vi "replace top level section in TOML data.vi"(7 "Section name":string caption="Section name (Section data name if empty)", 8 "error in (no error)":errorcluster, 10 "Section data":variant, 11 "Value in":T1) -> (0 "error out":errorcluster, 3 "Value out":T1)   [LabVIEW 2017, in "TOML.lvlib"]
doc: "Edit a top level element (section) in the TOML data\nMatch the elemnt by \"Section name\""
uses:
  TOML.lvlib
  TOML Value.ctl
  TOML Key-Value Pair.ctl
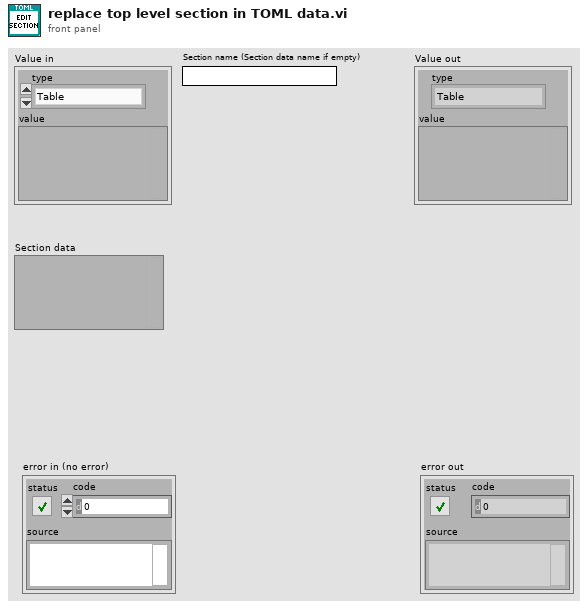
[diagram p1: front panel]
types:
  T1 = typedef "TOML.lvlib/TOML Value.ctl" = cluster{"type":enum16{"Table", "Array", "String", "Integer", "Float", "Boolean", "Offset Date-Time", "Local Date-Time", "Local Date", "Local Time", "Path"}, "value":variant}
  T2 = typedef "TOML.lvlib/TOML Key-Value Pair.ctl" = cluster{"Key":string, "Value":T1}
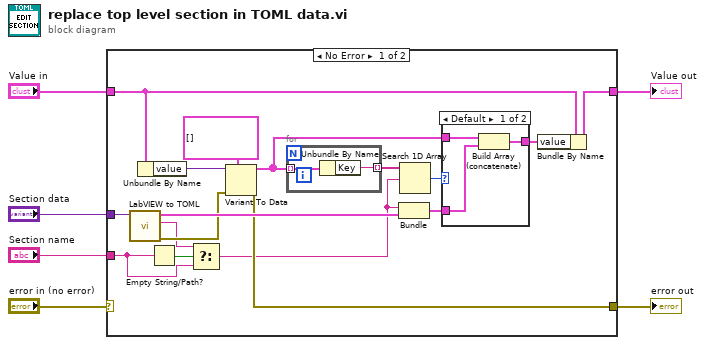
[diagram p0: block diagram]
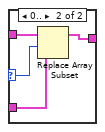
[diagram p2: hidden frame]
diagram:
  n1 = case shown="No Error" "error in (no error)" {
    selector: "error in (no error)" -> [_ w34]
    tunnel: [w22 w33] -> w6
    tunnel: "Value in" -> [w21 w33]
    tunnel: "Section data" -> [w13 _]
    tunnel: "Section name" -> [w8 _]
    tunnel: [w12 w34] -> w1
    frame No Error {
      n2 = call "LabVIEW to TOML.vi"("LV Value"=w13) -> ("error out"=w11:errorcluster, "Name"=w9:string, "TOML Value"=w19:T1)  [unwired: 8 in]
      n3 = Unbundle By Name(w21) -> ("value"=w20:variant)
      n4 = Empty String/Path?(string/path=w8) -> (empty?=w10:bool)
      n5 = Select(t=w9, s=w10, f=w8) -> (s? t:f=w7:string)
      n6 = Variant To Data(error in=w11, type=T2[] [], Variant=w20) -> (data=w16:T2[], error out=w12:errorcluster)
      n7 = for {
        tunnel: w16 -> [w32] mode=indexing
        tunnel: [w31] -> w17 mode=indexing
        n8 = Unbundle By Name(w32) -> ("Key"=w31:string)
      }
      n9 = Bundle("Section name"=w7, "TOML Value"=w19) -> (w15:cluster{"Section name":string, "TOML Value":T1})  [unwired: 1 in]
      n10 = Search 1D Array(1D array=w17, element=w7) -> (index of element=w14:i32)  [unwired: 1 in]
      n11 = case shown="Default" w14 {
        selector: w14 -> [_ w29]
        tunnel: w16 -> [w26 w30]
        tunnel: [w25 w28] -> w23
        tunnel: w15 -> [w24 w27]
        frame Default {
          n12 = Build Array (concatenate)(w26, w24) -> (w25:T2[])
        }
        frame 0.. {
          n13 = Replace Array Subset(array=w30, new element=w27, index=w29) -> (w28:T2[])
        }
      }
      n14 = Bundle By Name(cluster=w21, "value"=w23) -> (w22:T1)
    }
    frame Error {
    }
  }
  "Value out" <- w6
  "error out" <- w1
